vi "Build String Array w Max Size.vi"(6 "Max Size":i32=100, 7 "Initialize":bool, 10 "string":string) -> (2 "Array":string[](array[string]))   [LabVIEW 2009]
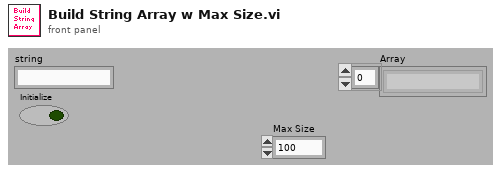
[diagram p1: front panel]
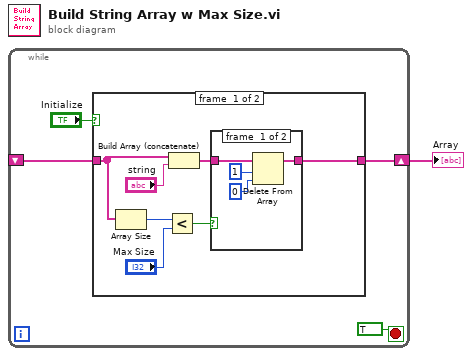
[diagram p0: block diagram]
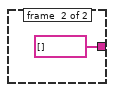
[diagram p3: hidden frame]
diagram:
  n1 = while {
    shift-right: [w4] -> w1
    shift-left: _ -> [w5]
    stop <- TRUE stop-if-true
    n2 = case shown="False" "Initialize" {
      tunnel: w5 -> [w11 _]
      tunnel: [w6 string[] []] -> w4
      frame #0 {
        n3 = Array Size(array=w11) -> (size(s)=w10:i32)
        n4 = Less?(x=w10, y="Max Size") -> (x < y?=w7:bool)
        n5 = Build Array (concatenate)(w11, "string") -> (w8:string[])
        n6 = case shown="True" w7 {
          tunnel: [w16 w17] -> w6
          tunnel: w8 -> [w15 w17]
          frame #0 {
            n7 = Delete From Array(array=w15, length=1, index=0) -> (array with subset deleted=w16:string[])  [unwired: 1 out]
          }
          frame #1 {
          }
        }
      }
      frame #1 {
      }
    }
  }
  "Array" <- w1
